vi "FTW-File-Directory-Exists.vi"(1 "Directory":path) -> (0 "Exists?":bool)   [LabVIEW 2012]
panel:
  # "Inputs"
  # "Outputs"
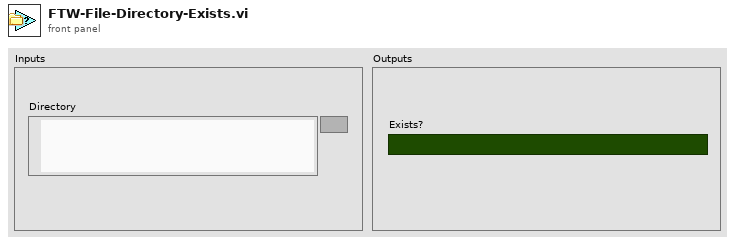
[diagram p1: front panel]
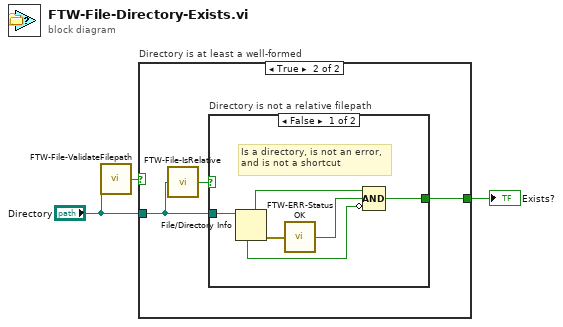
[diagram p0: block diagram]
diagram:
  n1 = call "FTW-File-ValidateFilepath.vi"("Filepath"="Directory") -> ("Valid?"=w1:bool)
  n2 = case "Directory is at least a well-formed" shown="True" w1 {
    tunnel: "Directory" -> [_ w5]
    tunnel: [_ w6] -> w3
    frame False {
    }
    frame True {
      n3 = call "FTW-File-IsRelative.vi"("Filepath"=w5) -> ("Relative?"=w4:bool)
      n4 = case "Directory is not a relative filepath" shown="False" w4 {
        tunnel: [w9 _] -> w6
        tunnel: w5 -> [w10 _]
        frame False {
          # "Is a directory, is not an error,\nand is not a shortcut"
          n5 = File/Directory Info(path=w10) -> (directory=w12:bool, error out=w8:errorcluster, shortcut=w11:bool)  [unwired: 1 in, 4 out]
          n6 = call "FTW-ERR-StatusOK.vi"("error to check"=w8) -> ("Status OK?"=w7:bool)
          n7 = Compound Arithmetic op=AND(w12, w7, invert w11) -> (w9:bool)
        }
        frame True {
        }
      }
    }
  }
  "Exists?" <- w3
